vi "Configuration Value Changed.vi"(8 "error in (no error)":errorcluster, 11 "Measure Object in":refnum<class "Template Module.lvclass">) -> (0 "error out":errorcluster, 3 "Measure Object out":refnum<class "Template Module.lvclass">)   [LabVIEW 2016, in "Template Module.lvclass"]
uses:
  Template Module.lvclass
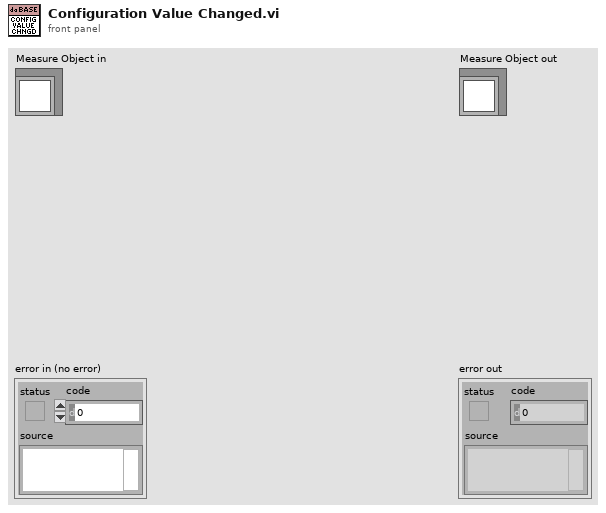
[diagram p1: front panel]
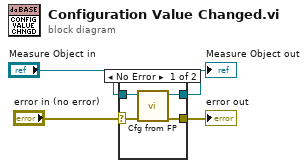
[diagram p0: block diagram]
diagram:
  n1 = case shown="No Error" "error in (no error)" {
    selector: "error in (no error)" -> [w8 w10]
    tunnel: [w7 w10] -> w3
    tunnel: [w5 w9] -> w1
    tunnel: "Measure Object in" -> [w6 w9]
    frame No Error {
      n2 = call-dynamic "Cfg from FP.vi"("error in (no error)"=w8, "Measure Object in"=w6) -> ("error out"=w7:errorcluster, "Measure Object out"=w5:refnum<class "Template Module.lvclass">)  [unwired: 8 in]
    }
    frame Error {
    }
  }
  "error out" <- w3
  "Measure Object out" <- w1
